vi "WaveformComponent, Append Leading Edge.vi"(0 "waveform in":waveform(dbl)={"t0"=timestamp(3474820848.0780005 s since 1904-01-01), "dt"=nan, "Y"=[]}, 1 "append parameters":T1={"offset"=0.5, "amplitude"=-2.0, "delay"=0.00019999999999999998, "leading edge"=0.0005, "pulse width"=0.0006, "trailing edge"=0.0005, "ref level %"=1.0} {"ref level %" format="%.3f"; "offset" format="%.3f"; "pulse width" format="%.1f"; "trailing edge" format="%.1f"; "amplitude" format="%.3f"; "delay" format="%.1f"; "leading edge" format="%.1f"}) -> (3 "waveform out":waveform(dbl)={"t0"=timestamp(-9593225999.921999 s since 1904-01-01), "dt"=nan, "Y"=[]})   [LabVIEW 2010]
uses:
  Pulse Parameters.ctl
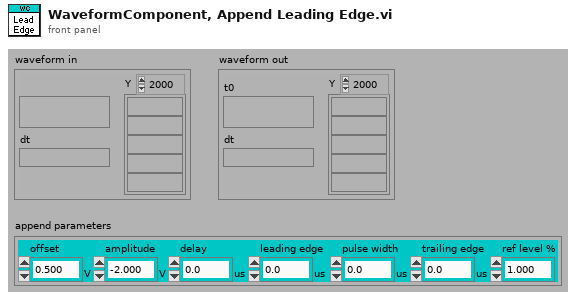
[diagram p1: front panel]
types:
  T1 = typedef "Pulse Parameters.ctl" = cluster{"offset":dbl[unit], "amplitude":dbl[unit], "delay":dbl[unit], "leading edge":dbl[unit], "pulse width":dbl[unit], "trailing edge":dbl[unit], "ref level %":dbl}
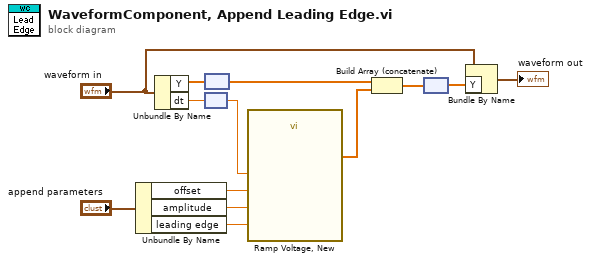
[diagram p0: block diagram]
diagram:
  n1 = Unbundle By Name("append parameters") -> ("offset"=w1:dbl[unit], "amplitude"=w2:dbl[unit], "leading edge"=w11:dbl[unit])
  n2 = Unbundle By Name("waveform in") -> ("Y"=w9:dbl[], "dt"=w7:dbl)
  n3 = node(w9) -> (w5:dbl[unit][])
  n4 = node(w7) -> (w6:dbl[unit])
  n5 = call "Ramp Voltage, New.vi"("offset (0.0)"=w1, "amplitude (0.0)"=w2, "dt"=w6, "total time"=w11) -> ("ramp"=w12:dbl[unit][])  [unwired: 1 in]
  n6 = Build Array (concatenate)(w5, w12) -> (w4:dbl[unit][])
  n7 = node(w4) -> (w13:dbl[])
  n8 = Bundle By Name(cluster="waveform in", "Y"=w13) -> (→"waveform out":waveform(dbl))
